vi "InitMultiThermal.vi"(8 "error in":errorcluster, 10 "I2C Addresses":u8[](array[numeric]), 11 "LINX Resource in":T2) -> (0 "error out":errorcluster, 1 "ThermalConfigs":T1(array[cluster]) {"I2C Slave Address" format="%.0x"}, 2 "ThermOnline":bool[](array[boolean]), 3 "LINX Resource out":T2)   [LabVIEW 2014]
uses:
  <vilib>/MakerHub/LINX/Private/Type Defs/LINX Ref.ctl
  <vilib>/MakerHub/LINX/Private/Type Defs/Platform.ctl
  <vilib>/MakerHub/LINX/Private/Type Defs/Interface.ctl
  <vilib>/MakerHub/LINX/Private/Device/Type Defs/LINX Device Config.ctl
  <vilib>/MakerHub/LINX/Private/Device/Type Defs/TCP Config.ctl
  <vilib>/MakerHub/LINX/Private/Device/Type Defs/Channels.ctl
  <vilib>/MakerHub/LINX/LMH-LINX.lvlib
  <vilib>/MakerHub/LINX/Private/Device/Device.lvlib
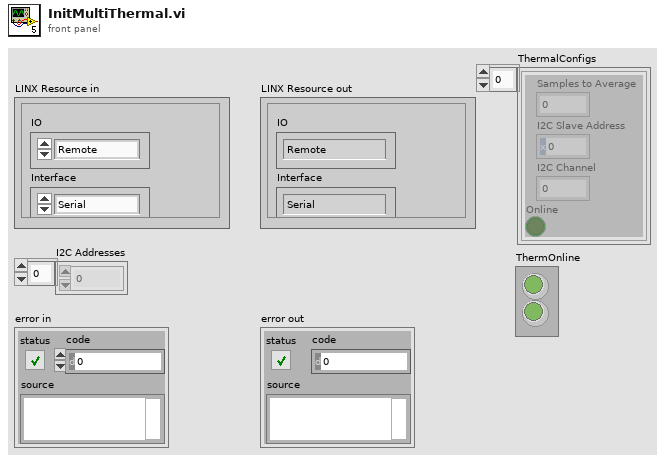
[diagram p1: front panel]
types:
  T1 = cluster{"Samples to Average":u16, "I2C Slave Address":u8, "I2C Channel":u8, "Online":bool}[]
  T2 = typedef "LMH-LINX.lvlib/LINX Ref.ctl" = cluster{"IO":T3, "Interface":T4, "LINX Device Config":T5}
  T3 = typedef "LMH-LINX.lvlib/Platform.ctl" = enum16{"Remote", "Local"}
  T4 = typedef "LMH-LINX.lvlib/Interface.ctl" = enum16{"Serial", "TCP"}
  T5 = typedef "LMH-LINX.lvlib/Device.lvlib/LINX Device Config.ctl" = cluster{"Interface":T4, "COM Port":refnum<visa-resource-name>, "TCP Configuration":T6, "Device Family":u8, "Device ID":u8, "Device Name":string, "TCP Ref":refnum<k5>, "Channels":T7}
  T6 = typedef "LMH-LINX.lvlib/Device.lvlib/TCP Config.ctl" = cluster{"IP Address":string, "Port":u16}
  T7 = typedef "LMH-LINX.lvlib/Channels.ctl" = cluster{"DI":u8[], "DO":u8[], "AI":u8[], "AO":u8[], "PWM":u8[], "QE":u8[], "UART":u8[], "I2C 2":u8[], "SPI":u8[], "CAN":u8[], "Servo":u8[], "AI Ref (V)":dbl, "AI Resolution (Bits)":u8, "AO Ref (V)":dbl, "AO Resolution (Bits)":u8}
  T8 = cluster{"Samples to Average":u16, "I2C Slave Address":u8, "I2C Channel":u8, "Online":bool}
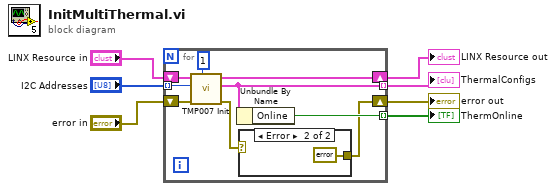
[diagram p0: block diagram]
diagram:
  n1 = for {
    shift-right: [w8] -> w4
    shift-left: "error in" -> [w16]
    shift-right: [w14] -> w6
    shift-left: "LINX Resource in" -> [w15]
    tunnel: "I2C Addresses" -> [w13] mode=indexing
    tunnel: [w11] -> w2 mode=indexing
    tunnel: [w10] -> w1 mode=indexing
    n2 = call "TMP007 Init.vi"("I2C Channel"=u8 1, "error in (no error)"=w16, "I2C Slave Address"=w13, "LINX Resource in"=w15) -> ("error out"=w9:errorcluster, "Thermopile Setting"=w11:T8, "LINX Resource out"=w14:T2)  [unwired: 5 in]
    n3 = Unbundle By Name(w11) -> ("Online"=w10:bool)
    n4 = case shown="Error" w9 {
      selector: w9 -> [w17 _]
      tunnel: [w17 errorcluster {"status"=FALSE, "code"=0, "source"=""} ("error in 2")] -> w8
      frame No Error {
      }
      frame Error {
      }
    }
  }
  "LINX Resource out" <- w6
  "error out" <- w4
  "ThermalConfigs" <- w2
  "ThermOnline" <- w1
